vi "Force Tester.vi"() -> ()   [LabVIEW 2020]
uses:
  <vilib>/DAQmx/read.llb/DAQmx Read (Analog 1D DBL 1Chan NSamp).vi
  <vilib>/DAQmx/create/channels.llb/DAQmx Create Channel (AI-Voltage-Basic).vi
  <vilib>/DAQmx/configure/timing.llb/DAQmx Timing (Sample Clock).vi
  <vilib>/DAQmx/miscellaneous.llb/DAQmx Fill In Error Info.vi
panel:
  out "force data":cluster{i32[], dbl[]}(graph)
  in  "stop":bool
  out "force (V)":dbl
  in  "freq":dbl=1000.0 format="%0.2f"
  in  "physical channels":tag
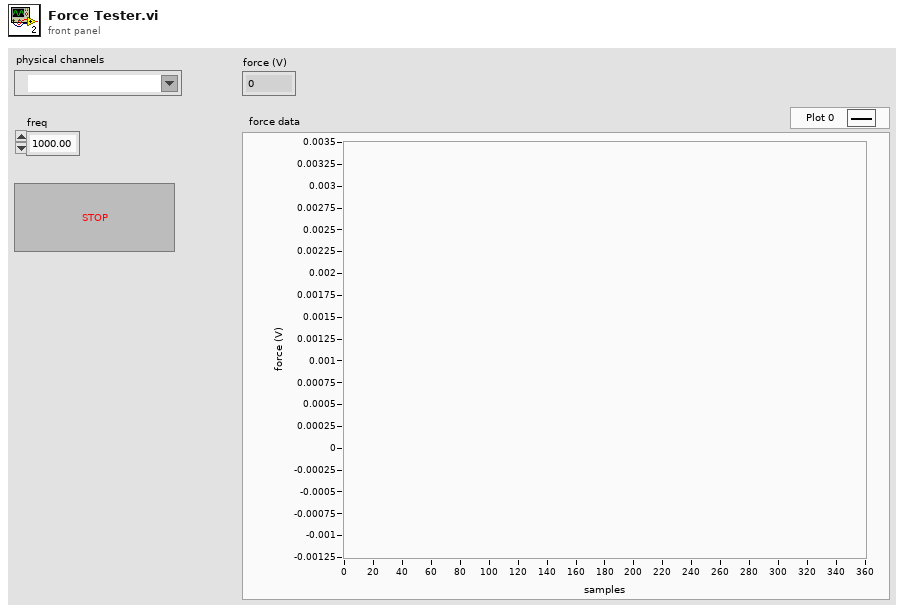
[diagram p1: front panel]
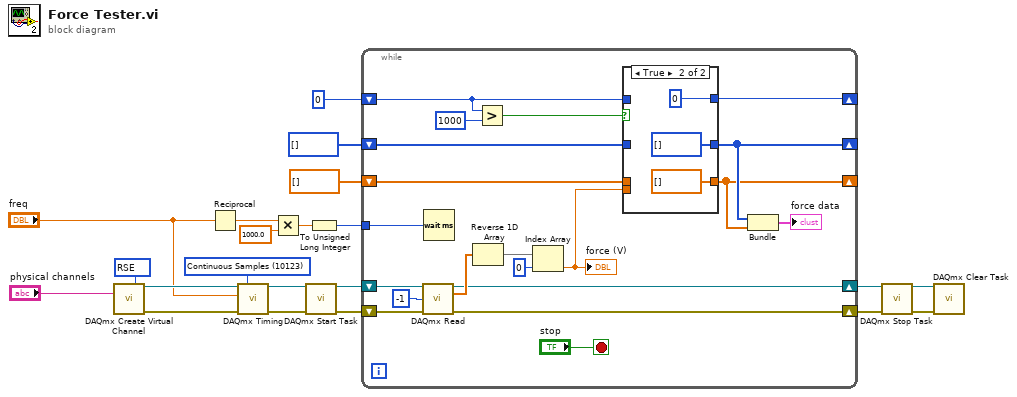
[diagram p0: block diagram]
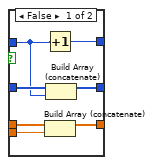
[diagram p2: hidden frame]
diagram:
  w19 = 10083 items=["Default"=-1, "RSE"=10083, "NRSE"=10078, "Differential"=10106, "Pseudodifferential"=12529] ("input terminal configuration")
  w18 = 10123 items=["Finite Samples"=10178, "Continuous Samples"=10123, "Hardware Timed Single Point"=12522] ("sample mode")
  n1 = call-poly <vilib>:"DAQmx Create Virtual Channel.vi"("input terminal configuration"=w19, "physical channels"="physical channels") -> ("task out"=w20:refnum<k21>, "error out"=w21:errorcluster)  [unwired: 12 in]
  n2 = Reciprocal(x="freq") -> (1/x=w4:dbl)
  n3 = call-poly <vilib>:"DAQmx Timing.vi"("task/channels in"=w20, "sample mode"=w18, "rate"="freq", "error in"=w21) -> ("task out"=w16:refnum<k21>, "error out"=w17:errorcluster)  [unwired: 10 in]
  n4 = Multiply(x=w4, y=1000.0) -> (x*y=w2:dbl)
  n5 = call <vilib>:"DAQmx Start Task.vi"("task/channels in"=w16, "error in"=w17) -> ("task out"=w13:refnum<k21>, "error out"=w14:errorcluster)  [unwired: 12 in]
  n6 = To Unsigned Long Integer(number=w2) -> (unsigned 32bit integer=w1:u32)
  n7 = while {
    shift-right: [w35] -> w10
    shift-left: w14 -> [w37]
    shift-right: [w34] -> w9
    shift-left: w13 -> [w36]
    shift-right: [w29] -> _
    shift-left: 0 -> [w30]
    shift-right: [w24] -> _
    shift-left: dbl[] [] ("reversed array") -> [w28]
    shift-right: [w25] -> _
    shift-left: i32[] [] -> [w26]
    tunnel: w1 -> [w22]
    stop <- "stop" stop-if-true
    n8 = call-poly <vilib>:"DAQmx Read.vi"("task/channels in"=w36, "number of samples per channel"=-1, "error in"=w37) -> ("task out"=w34:refnum<k21>, "data"=w41:dbl[], "error out"=w35:errorcluster)  [unwired: 10 in]
    n9 = Wait (ms)(milliseconds to wait=w22) -> ()  [unwired: 1 out]
    n10 = Reverse 1D Array(array=w41) -> (reversed array=w40:dbl[])
    n11 = Greater?(x=w30, y=1000) -> (0:w31:bool)
    n12 = Index Array ("Take most recent data point")(array=w40, index=0) -> (element=w27:dbl)
    "force (V)" <- w27
    n13 = case shown="True" w31 {
      tunnel: w30 -> [w43 _]
      tunnel: [w48 0] -> w29
      tunnel: w28 -> [w47 _]
      tunnel: w27 -> [w46 _]
      tunnel: [w45 dbl[] []] -> w24
      tunnel: w26 -> [w44 _]
      tunnel: [w42 i32[] []] -> w25
      frame False {
        n14 = Increment(x=w43) -> (x+1=w48:i32)
        n15 = Build Array (concatenate)(w47, w46) -> (w45:dbl[])
        n16 = Build Array (concatenate)(w44, w43) -> (w42:i32[])
      }
      frame True {
      }
    }
    n17 = Bundle(w25, w24) -> (→"force data":cluster{i32[], dbl[]})  [unwired: 1 in]
  }
  n18 = call <vilib>:"DAQmx Stop Task.vi"("task/channels in"=w9, "error in"=w10) -> ("task out"=w11:refnum<k21>, "error out"=w12:errorcluster)  [unwired: 12 in]
  n19 = call <vilib>:"DAQmx Clear Task.vi"("task in"=w11, "error in"=w12) -> ()  [unwired: 13 in, 1 out]
